vi "MasterRobotModeController.vi"() -> (1 "FMS Robot Mode":T1, 2 "Auto Reset":bool, 3 "Robot is Autonomous":bool)   [LabVIEW 2020]
doc: "This state controller manages the Robot Mode and whether or not the robot is running autonomously. The robot will continue running autonomously after Autonomous Mode ends, until the driver touches the joystick during TeleOperated Mode or until/unless the FORCE HUMAN CONTROL override is flipped on the FRC 4265 Dashboard."
uses:
  <vilib>/Rock Robotics/WPI/DriverStation/WPI_DriverStationRobotMode2.ctl
  GlobalDriverStationData.vi
  robotconstants.vi
  GlobalDriverStationCommands.vi
  GRNF_Joystick.vi
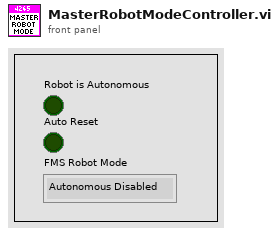
[diagram p1: front panel]
types:
  T1 = typedef "WPI_DriverStationRobotMode2.ctl" = enum16{"Autonomous Disabled", "Autonomous Enabled", "Teleop Disabled", "Teleop Enabled", "Disconnected", "Finish", "Test Disabled", "Test Enabled", "Emergency Stopped"}
  T2 = typedef "WPI_JoystickDevRef.ctl" = cluster{"Device":T3}
  T3 = typedef "WPI_JoystickDeviceEnum.ctl" = enum16{"USB 0", "USB 1", "USB 2", "USB 3", "USB 4", "USB 5"}
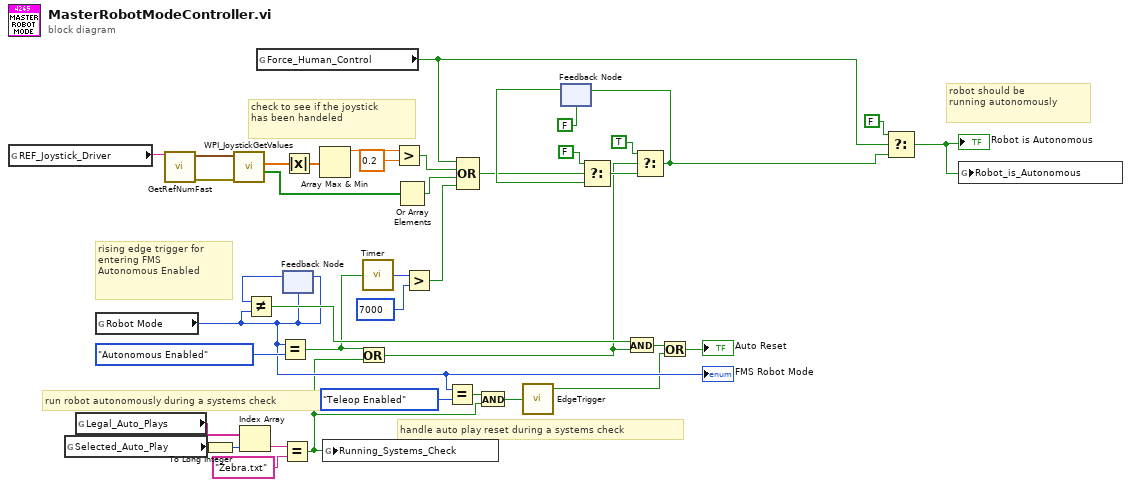
[diagram p0: block diagram]
diagram:
  # "handle auto play reset during a systems check"
  # "run robot autonomously during a systems check"
  # "rising edge trigger for\nentering FMS\nAutonomous Enabled"
  # "robot should be\nrunning autonomously"
  # "check to see if the joystick \nhas been handeled"
  n1 = global read "GlobalDriverStationCommands.vi" "REF_Joystick_Driver"() -> (w1:string)
  n2 = global read "GlobalDriverStationData.vi" "Selected_Auto_Play"() -> (w15:u16)
  n3 = global read "robotconstants.vi" "Legal_Auto_Plays"() -> (w10:string[])
  n4 = global read "GlobalDriverStationData.vi" "Robot Mode"() -> (w6:T1)
  "FMS Robot Mode" <- w6
  n5 = call-poly "GetRefNumFast.vi"("RefNum Name"=w1) -> ("Error"=w40:errorcluster, "Device Reference"=w41:T2)  [unwired: 5 in]
  n6 = To Long Integer(number=w15) -> (32bit integer=w16:i32)
  n7 = call <vilib>:"WPI_JoystickGetValues.vi"("error in (no error)"=w40, "JoystickDevRef"=w41) -> ("Buttons"=w39:bool[], "Axes"=w38:dbl[])  [unwired: 5 in, 3 out]
  n8 = Index Array(array=w10, index=w16) -> (element=w14:string)
  n9 = global read "GlobalDriverStationData.vi" "Force_Human_Control"() -> (w20:bool)
  n10 = Equal?(x=w6, y=WPI_DriverStationRobotMode2."Autonomous Enabled" ("Robot Mode")) -> (x = y?=w11:bool)
  n11 = Equal?(x=w14, y="Zebra.txt") -> (x = y?=w4:bool)
  n12 = feedback #1(w6) -> (w29:T1)
  n13 = Not Equal?(x=w29, y=w6) -> (x != y?=w28:bool)
  n14 = feedback-in #1(w6) -> ()
  n15 = Absolute Value(x=w38) -> (abs(x)=w37:dbl[])
  n16 = Array Max & Min(array=w37) -> (max value=w36:dbl)  [unwired: 3 out]
  n17 = global write "GlobalDriverStationData.vi" "Running_Systems_Check"(w4) -> ()
  n18 = Or(x=w11, y=w4) -> (x .or. y?=w12:bool)
  n19 = call "Timer.vi"("Reset Timer"=w11) -> ("Time (ms)"=w19:u32)
  n20 = Greater?(x=w36, y=0.2) -> (0:w34:bool)
  n21 = Or Array Elements(Boolean array=w39) -> (logical OR=w33:bool)
  n22 = Greater?(x=w19, y=u32 7000) -> (0:w17:bool)
  n23 = Equal?(x=w6, y=WPI_DriverStationRobotMode2."Teleop Enabled" ("Robot Mode")) -> (x = y?=w5:bool)
  n24 = Compound Arithmetic op=OR(w20, w34, w33, w17) -> (w24:bool)
  n25 = And(x=w5, y=w4) -> (x .and. y?=w3:bool)
  n26 = call "EdgeTrigger.vi"("Input Signal"=w3) -> ("Rising Edge Trigger"=w2:bool)  [unwired: 2 out]
  n27 = feedback #2(FALSE) -> (w25:bool)
  n28 = Select(t=FALSE, s=w24, f=w25) -> (s? t:f=w26:bool)
  n29 = And(x=w28, y=w12) -> (x .and. y?=w9:bool)
  n30 = Select(t=TRUE, s=w12, f=w26) -> (s? t:f=w22:bool)
  n31 = feedback-in #2(w22) -> ()
  n32 = Or(x=w9, y=w2) -> (x .or. y?=→"Auto Reset":bool)
  n33 = Select(t=FALSE, s=w20, f=w22) -> (s? t:f=w21:bool)
  "Robot is Autonomous" <- w21
  n34 = global write "GlobalDriverStationData.vi" "Robot_is_Autonomous"(w21) -> ()
